vi "Scale and Wrap Attitude.vi"(10 "draw options":T2={"Text Color"=16777238, "Wing Color"=16751616, "Dial Outline Color"=13816530, "Sky Color"=3381759, "Ground Color"=8213043, "Horizon Line Color"=16777225, "Outline Color"=0, "Dial Background Color"=5987163, "Draw Wings"=TRUE, "Draw Text"=TRUE, "Font Name"="Helvetica", "Angle units"=enum."Degrees"}, 11 "attitude":T1) -> (3 "attitude (rad)":T1)   [LabVIEW 2017, in "NI_Robotics_Attitude Picture.lvlib"]
uses:
  <vilib>/robotics/Controls/Attitude Indicator/Attitude Picture/NI_Robotics_Attitude Picture.lvlib
  <vilib>/robotics/Controls/Attitude Indicator/Attitude Picture/Attitude.ctl
  <vilib>/robotics/Controls/Attitude Indicator/Attitude Picture/Draw Options.ctl
  <vilib>/robotics/Controls/Utilities/Angle Units.ctl
  <vilib>/Analysis/coordinate.llb/Angle Range (Degree).ctl
  <vilib>/Analysis/coordinate.llb/Angle Units.ctl
  <vilib>/Analysis/coordinate.llb/Wrap Angle (scalar).vi
  <vilib>/Utility/AngleManip/Degrees to Radians (Scalar DBL).vi
  <vilib>/Analysis/NI_AAL_Angle.lvlib
  <vilib>/Utility/AngleManip/NI_AngleManipulation.lvlib
  <vilib>/robotics/Controls/Utilities/NI_Robotics_Control Utilities.lvlib
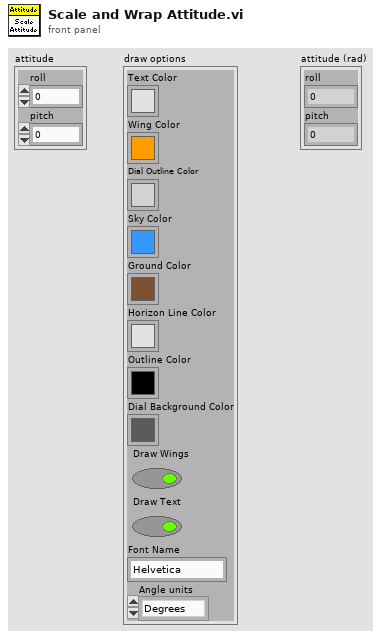
[diagram p1: front panel]
types:
  T1 = typedef "NI_Robotics_Attitude Picture.lvlib/Attitude.ctl" = cluster{"roll":dbl, "pitch":dbl}
  T2 = typedef "NI_Robotics_Attitude Picture.lvlib/Draw Options.ctl" = cluster{"Text Color":u32, "Wing Color":u32, "Dial Outline Color":u32, "Sky Color":u32, "Ground Color":u32, "Horizon Line Color":u32, "Outline Color":u32, "Dial Background Color":u32, "Draw Wings":bool, "Draw Text":bool, "Font Name":string, "Angle units":T3}
  T3 = typedef "NI_Robotics_Control Utilities.lvlib/Angle Units.ctl" = enum16{"Radians", "Degrees"}
  T4 = typedef "NI_AAL_Angle.lvlib/Angle Units.ctl" = i32
  T5 = typedef "NI_AAL_Angle.lvlib/Angle Range (Degree).ctl" = u16
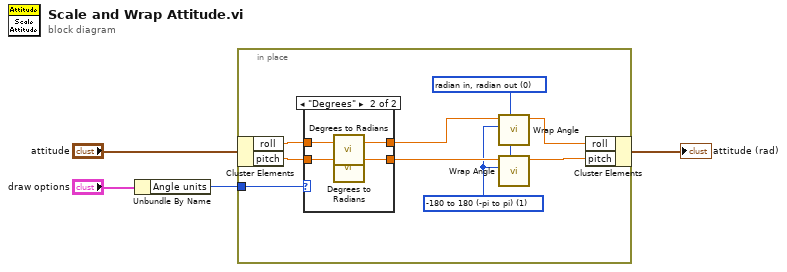
[diagram p0: block diagram]
diagram:
  n1 = Unbundle By Name("draw options") -> ("Angle units"=w1:T3)
  n2 = in-place {
    in-place-border: w1 -> [w11]
    w6 = T4 0 items=["radian in, radian out", "radian in, degree out", "degree in, degree out", "degree in, radian out"] ("angle units")
    w5 = T5 1 items=["none", "-180 to 180 (-pi to pi)", "0 to 360 (0 to 2pi)"] ("angle range")
    n3 = in-place-cluster #1("attitude") -> ("roll"=w13:dbl, "pitch"=w12:dbl)
    n4 = case shown="\"Degrees\"" w11 {
      tunnel: w13 -> [w15 w19]
      tunnel: [w15 w18] -> w7
      tunnel: [w14 w17] -> w9
      tunnel: w12 -> [w14 w16]
      frame "Radians", Default {
      }
      frame "Degrees" {
        n5 = call-poly <vilib>:"Degrees to Radians.vi"("angle (deg)"=w19) -> ("angle (rad)"=w18:dbl)  [unwired: 2 in]
        n6 = call-poly <vilib>:"Degrees to Radians.vi"("angle (deg)"=w16) -> ("angle (rad)"=w17:dbl)  [unwired: 2 in]
      }
    }
    n7 = call-poly <vilib>:"Wrap Angle.vi"("angle units"=w6, "angle range"=w5, "angle in"=w7) -> ("angle out"=w8:dbl)  [unwired: 7 in, 1 out]
    n8 = call-poly <vilib>:"Wrap Angle.vi"("angle units"=w6, "angle range"=w5, "angle in"=w9) -> ("angle out"=w10:dbl)  [unwired: 7 in, 1 out]
    n9 = in-place-cluster #1("roll"=w8, "pitch"=w10) -> (→"attitude (rad)":T1)
  }
